vi "Write AllowUserToDeleteRows.vi"(8 "error in (no error)":errorcluster, 10 "AllowUserToDeleteRows":bool, 11 "DataGridView in":refnum<class "DataGridView.lvclass">) -> (0 "error out":errorcluster, 3 "DataGridView out":refnum<class "DataGridView.lvclass">)   [LabVIEW 2013, in "DataGrid.lvlib" / "DataGridView.lvclass"]
uses:
  DataGridView.lvclass
  DataGridView.lvclass/DataGridView.ctl
  System.Windows.Forms
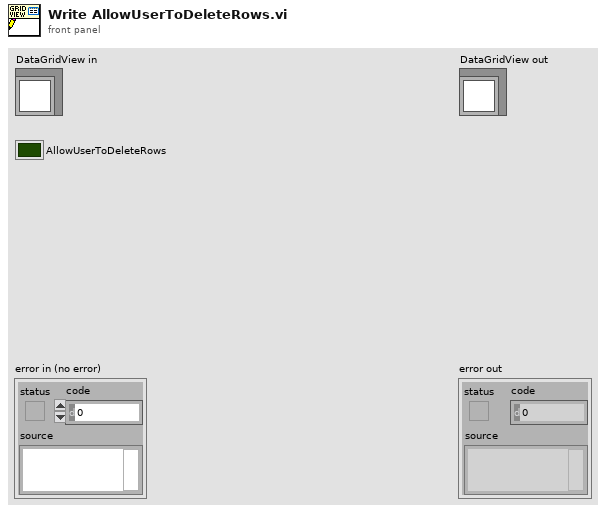
[diagram p1: front panel]
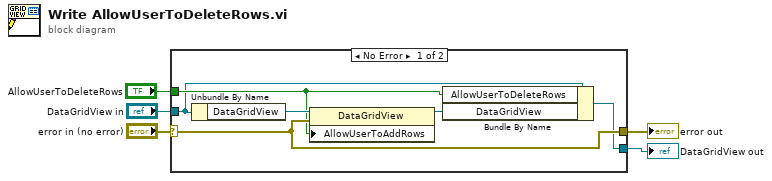
[diagram p0: block diagram]
diagram:
  n1 = case shown="No Error" "error in (no error)" {
    selector: "error in (no error)" -> [w11 w12]
    tunnel: [w11 w12] -> w4
    tunnel: [w10 w13] -> w2
    tunnel: "DataGridView in" -> [w6 w13]
    tunnel: "AllowUserToDeleteRows" -> [w7 _]
    frame No Error {
      n2 = Unbundle By Name(w6) -> ("DataGridView"=w9:refnum<k24>)
      n3 = property class="DataGridView"(reference=w9, error in=w11, "AllowUserToAddRows"=w7) -> (reference out=w8:refnum<k24>)  [unwired: 1 out]
      n4 = Bundle By Name(cluster=w6, "AllowUserToDeleteRows"=w7, "DataGridView"=w8) -> (w10:refnum<class "DataGridView.lvclass">)
    }
    frame Error {
    }
  }
  "error out" <- w4
  "DataGridView out" <- w2
